vi "Validate JSON file.vi"(8 "error in (no error)":errorcluster, 11 "json file":path) -> (0 "error out":errorcluster)   [LabVIEW 2017]
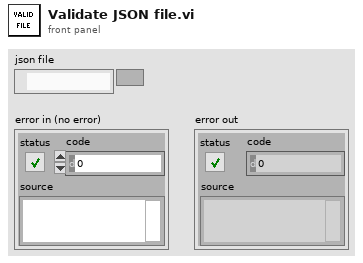
[diagram p1: front panel]
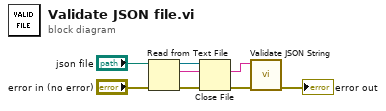
[diagram p0: block diagram]
diagram:
  n1 = Read from Text File(file (use dialog)="json file", error in="error in (no error)") -> (refnum out=w1:refnum<file>, text=w6:string, error out=w3:errorcluster)  [unwired: 2 in, 1 out]
  n2 = Close File(refnum=w1, error in=w3) -> (error out=w2:errorcluster)  [unwired: 1 out]
  n3 = call "Validate JSON String.vi"("error in (no error)"=w2, "String"=w6) -> ("error out"=→"error out":errorcluster)  [unwired: 8 in, 1 out]
